vi "FlatToRichcif_manager_QueryPluginLoadersRequest.vi"(5 "OutputClusterType":T1, 11 "InputCluster":T2) -> (3 "OutputCluster":T1)   [LabVIEW 2021, in "CIF_PluginLoader_client.lvlib"]
uses:
  cif_manager_QueryPluginLoadersRequest_Flat.ctl
  cif_manager_QueryPluginLoadersRequest.ctl
  CIF_PluginLoader_client.lvlib
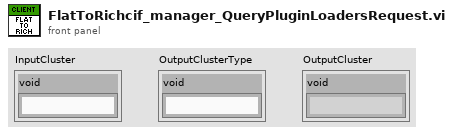
[diagram p1: front panel]
types:
  T1 = typedef "CIF_PluginLoader_client.lvlib/cif_manager_QueryPluginLoadersRequest.ctl" = cluster{"void":string}
  T2 = typedef "CIF_PluginLoader_client.lvlib/cif_manager_QueryPluginLoadersRequest_Flat.ctl" = cluster{"void":string}
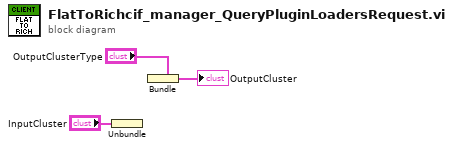
[diagram p0: block diagram]
diagram:
  n1 = Unbundle "Unbundle"("InputCluster") -> ()  [unwired: 1 out]
  n2 = Bundle "Bundle"(cluster="OutputClusterType") -> (→"OutputCluster":T1)  [unwired: 1 in]
